vi "ListFiles.vi"(0 "root directory":path, 5 "enter llbs? (no)":bool, 7 "pattern (none)":string, 11 "error in (no error)":errorcluster) -> (4 "dup root":path, 8 "file list":path[](array[path]), 15 "error out":errorcluster)   [LabVIEW 2011]
doc: "Recursively lists the files contained in a root directory. Optionally, the content of VI libraries can also be listed."
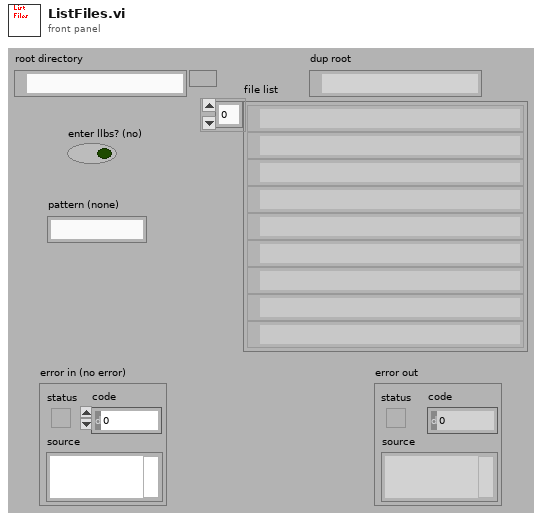
[diagram p1: front panel]
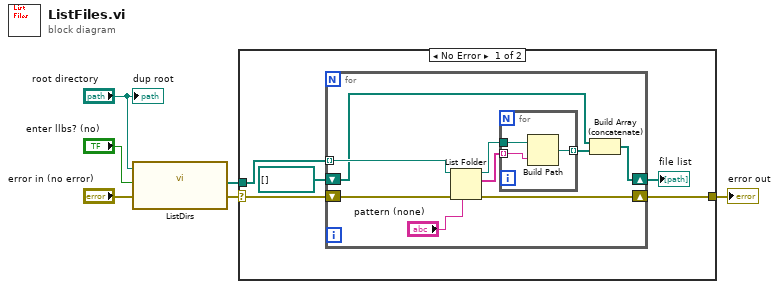
[diagram p0: block diagram]
diagram:
  n1 = call "ListDirs.vi"("root directory"="root directory", "include llbs? (no)"="enter llbs? (no)", "error in (no error)"="error in (no error)") -> ("directory/llb list, including root"=w3:path[], "error out"=w4:errorcluster)  [unwired: 10 in, 1 out]
  n2 = case shown="No Error" w4 {
    selector: w4 -> [w10 w24]
    tunnel: [w7 w24] -> w6
    tunnel: w3 -> [w11 _]
    frame No Error {
      n3 = for {
        tunnel: w11 -> [w20] mode=indexing
        shift-right: [w17] -> w7
        shift-left: w10 -> [w19]
        shift-right: [w12] -> w8
        shift-left: path[] [] ("directory list, including root") -> [w13]
        n4 = List Folder(path=w20, pattern="pattern (none)", error in=w19) -> (path out=w15:path, filenames=w16:string[], error out=w17:errorcluster)  [unwired: 1 in, 1 out]
        n5 = for {
          tunnel: w16 -> [w22] mode=indexing
          tunnel: w15 -> [w23]
          tunnel: [w21] -> w14 mode=indexing
          n6 = Build Path(base path=w23, name or relative path=w22) -> (appended path=w21:path)
        }
        n7 = Build Array (concatenate)(w13, w14) -> (w12:path[])
      }
      "file list" <- w8
    }
    frame Error {
    }
  }
  "error out" <- w6
  "dup root" <- "root directory"
